vi "cvi_generate_log_lags.vi"(8 "error in (no error)":errorcluster, 10 "coarseness":dbl=8.0 format="%#_13g", 11 "t_end":dbl=100000000000000.0 format="%#_13g") -> (0 "error out":errorcluster, 1 "division_factor":dbl[](array[numeric]), 2 "lag_bin_centers":dbl[](array[numeric]), 3 "lag_bins":dbl[](array[numeric]), 5 "num_lags":i32)   [LabVIEW 2015]
uses:
  cvibuild.corr_funcs/Release/corr_funcs.dll
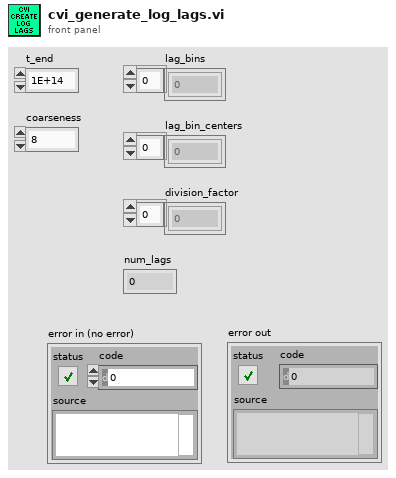
[diagram p1: front panel]
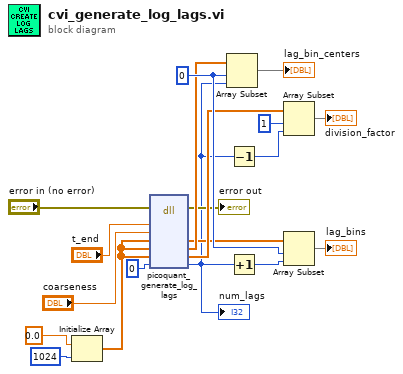
[diagram p0: block diagram]
diagram:
  w18 = 0 ("index")
  n1 = Initialize Array(0.0 ("element"), 1024 ("dimension size")) -> (w10:dbl[])
  n2 = dll-call lib="C:/Users/bspoka/Downloads/lvoop_dll-master/cvi_project/cvibuild.corr_funcs/Release/corr_funcs.dll" fn="picoquant_generate_log_lags"(error in="error in (no error)", "t_end"="t_end", "coarseness"="coarseness", "lag_bin_edges"=w10, "lags"=w10, "division_factor"=w10, "num_lags"=0) -> (error out=→"error out":errorcluster, "lag_bin_edges"=w12:dbl[], "lags"=w13:dbl[], "division_factor"=w17:dbl[], "num_lags"=w2:i32)  [unwired: 5 in, 1 out]
  "num_lags" <- w2
  n3 = Array Subset(array=w13, index=w18, length=w2) -> (→"lag_bin_centers":dbl[])
  n4 = Decrement(x=w2) -> (x-1=w1:i32)
  n5 = Increment(x=w2) -> (x+1=w14:i32)
  n6 = Array Subset(array=w17, index=1, length=w1) -> (→"division_factor":dbl[])
  n7 = Array Subset(array=w12, index=w18, length=w14) -> (→"lag_bins":dbl[])
